vi "RotationalPID.vi"(7 "Rotational PID Gains":T2={"proportional gain (Kc)"=1.0, "integral gain"=0.0, "derivative gain"=0.0} {"derivative gain" min=-0.1 max=0.1 step=1e-05 format="%.5f"; "integral gain" min=-10.0 max=10.0 step=1e-05 format="%.5f"; "proportional gain (Kc)" format="%.3f"}, 8 "Old Error [radians]":dbl=0.3418962909212272, 9 "Old Integral Error [radians*ms]":dbl=-10.0, 10 "dTime [ms]":dbl, 11 "DistanceToTarget [pixels]":T1) -> (0 "New Error [radians]":dbl=0.3349656440855023, 1 "New Integral Error [radians*ms]":dbl=-1.0, 3 "Spin Fraction Response":dbl=0.013384764469748641)   [LabVIEW 2018]
panel:
  in  "Image PPI [Pixels/Inch]":dbl=212.0
  in  "Length of Camera Boom [inches]":dbl=8.0
  # "RotationalPID"
  # "This class takes in the distance to the target and from that generates a rotational response which is coerced to be within [-1,1].\n\nIt calculates the angle from the positive y axis to the tracking target about the origin (robot's point of rotation) and uses this angle as the error.\n\nIt ouputs a New Error which is intended to be fed into the this VI during the next execution.\n\nThe Measured PPI is currently 212ppi and the current boom length is 8\"  These values were attained empirically, by measuring the camera's FOV on the ground and by measuring the camera boom length\n\nThis VI also zeros the Derivative and Integral responses when the tracking target  is lost (when \"Object Aquired\" is false)."
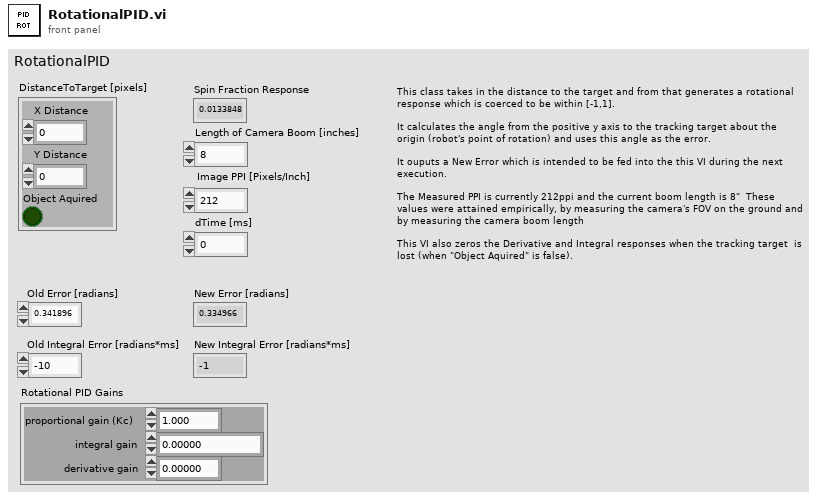
[diagram p1: front panel]
types:
  T1 = cluster{"X Distance":i32, "Y Distance":i32, "Object Aquired":bool}
  T2 = cluster{"proportional gain (Kc)":dbl, "integral gain":dbl, "derivative gain":dbl}
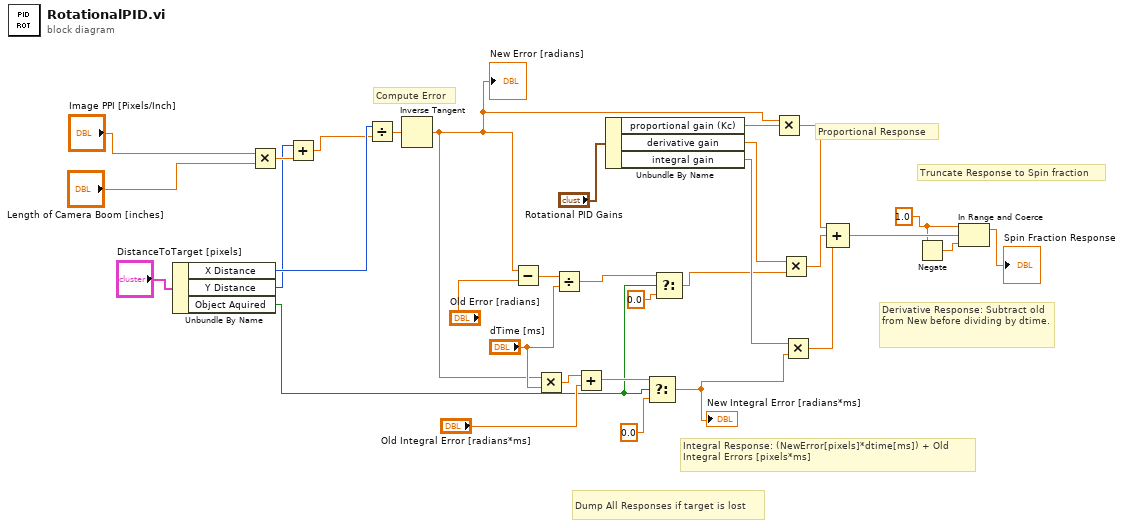
[diagram p0: block diagram]
diagram:
  w13 = 1.0 ("upper limit")
  # "Dump All Responses if target is lost"
  # "Truncate Response to Spin fraction"
  # "Derivative Response: Subtract old from New before dividing by dtime."
  # "Integral Response: (NewError[pixels]*dtime[ms]) + Old Integral Errors [pixels*ms]"
  # "Proportional Response"
  # "Compute Error"
  n1 = Unbundle By Name("DistanceToTarget [pixels]") -> ("X Distance"=w31:i32, "Y Distance"=w6:i32, "Object Aquired"=w3:bool)
  n2 = Multiply(x="Image PPI [Pixels/Inch]", y="Length of Camera Boom [inches]") -> (x*y=w25:dbl)
  n3 = Add(x=w6, y=w25) -> (x+y=w26:dbl)
  n4 = Divide(x=w31, y=w26) -> (x/y=w30:dbl)
  n5 = Inverse Tangent(1:w30) -> (0:w10:dbl)
  "New Error [radians]" <- w10
  n6 = Subtract(x=w10, y="Old Error [radians]") -> (x-y=w18:dbl)
  n7 = Multiply(x=w10, y="dTime [ms]") -> (x*y=w20:dbl)
  n8 = Divide(x=w18, y="dTime [ms]") -> (x/y=w2:dbl)
  n9 = Add(x=w20, y="Old Integral Error [radians*ms]") -> (x+y=w7:dbl)
  n10 = Unbundle By Name("Rotational PID Gains") -> ("proportional gain (Kc)"=w22:dbl, "derivative gain"=w12:dbl, "integral gain"=w16:dbl)
  n11 = Select(t=w7, s=w3, f=0.0) -> (s? t:f=w8:dbl)
  "New Integral Error [radians*ms]" <- w8
  n12 = Select(t=w2, s=w3, f=0.0) -> (s? t:f=w1:dbl)
  n13 = Multiply(x=w10, y=w22) -> (x*y=w11:dbl)
  n14 = Multiply(x=w12, y=w1) -> (x*y=w21:dbl)
  n15 = Multiply(x=w16, y=w8) -> (x*y=w19:dbl)
  n16 = Compound Arithmetic op=ADD(w11, w21, w19) -> (w28:dbl)
  n17 = Negate(x=w13) -> (-x=w14:dbl)
  n18 = In Range and Coerce(upper limit=w13, x=w28, lower limit=w14) -> (coerced(x)=→"Spin Fraction Response":dbl)  [unwired: 1 out]
